vi "Initiate.vi"(8 "error in (no error)":errorcluster, 11 "NI Scope in":refnum<class "NI Scope.lvclass">) -> (0 "error out":errorcluster, 3 "NI Scope out":refnum<class "NI Scope.lvclass">)   [LabVIEW 2025, in "Scope.lvlib" / "NI Scope.lvclass"]
uses:
  NI Scope.lvclass
  NI Scope.lvclass/NI Scope.ctl
  Scope Instrument/Scope Instrument.lvclass
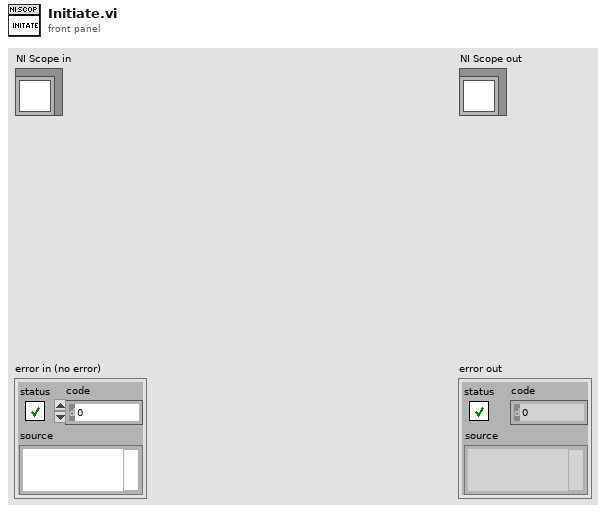
[diagram p1: front panel]
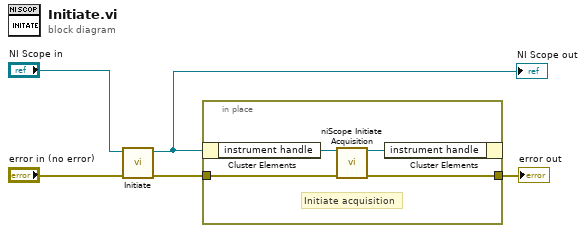
[diagram p0: block diagram]
diagram:
  n1 = call-parent "Initiate.vi"("error in (no error)"="error in (no error)", "Scope Instrument in"="NI Scope in") -> ("error out"=w3:errorcluster, "Scope Instrument out"=w1:refnum<class "NI Scope.lvclass">)  [unwired: 8 in]
  "NI Scope out" <- w1
  n2 = in-place {
    in-place-border: w3 -> [w9]
    in-place-border: [w8] -> w2
    # "Initiate acquisition"
    n3 = in-place-cluster #1(w1) -> ("instrument handle"=w7:refnum<k15>)
    n4 = call <instrlib>:"niScope Initiate Acquisition.vi"("instrument handle"=w7, "error in"=w9) -> ("instrument handle out"=w6:refnum<k15>, "error out"=w8:errorcluster)  [unwired: 12 in]
    n5 = in-place-cluster #1("instrument handle"=w6) -> ()  [unwired: 1 out]
  }
  "error out" <- w2
